vi "Logging2File.vi"(0 "log":string) -> (1 "LogFilePath":path, 2 "TimedLog":string)   [LabVIEW 2020]
doc: "Write to Log file and Send message to message window.\nLogs: .\\logs\\txt\nmessage: main.vi\\msg"
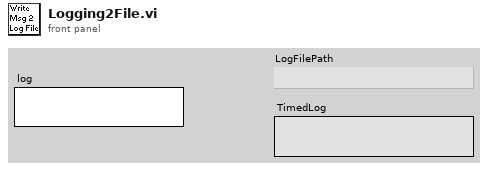
[diagram p1: front panel]
types:
  T1 = enum16{"open", "replace", "create", "open or create", "replace or create", "replace or create with confirmation"}
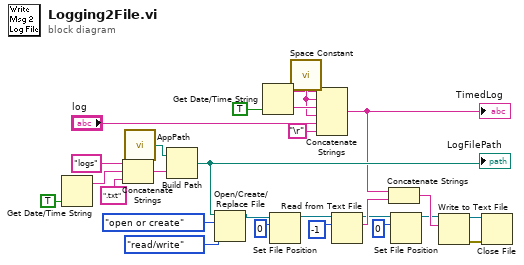
[diagram p0: block diagram]
diagram:
  n1 = Get Date/Time String(want seconds? (F)=TRUE) -> (date string=w24:string)  [unwired: 3 out]
  n2 = Concatenate Strings("logs" ("string"), w24, ".txt" ("string")) -> (w21:string)
  n3 = call "AppPath.vi"() -> ("AppPath"=w19:path)
  n4 = Build Path(base path=w19, name or relative path=w21) -> (appended path=w20:path)
  "LogFilePath" <- w20
  n5 = Open/Create/Replace File(file path (use dialog)=w20, operation (0:open)=T1."open or create", access (0:read/write)=enum16{"read/write", "read-only", "write-only"}."read/write") -> (refnum out=w1:refnum<file>)  [unwired: 1 in, 4 out]
  n6 = Get Date/Time String(want seconds? (F)=TRUE) -> (date string=w15:string, time string=w18:string)  [unwired: 2 out]
  n7 = Set File Position(offset (in bytes) (0)=i64 0, refnum=w1) -> (refnum out=w9:refnum<file>)  [unwired: 2 in, 1 out]
  n8 = call <vilib>:"Space Constant.vi"() -> ("String"=w17:string)
  n9 = Concatenate Strings(w15, w17, w18, w17, "log", "\r") -> (w4:string)
  "TimedLog" <- w4
  n10 = Read from Text File(file (use dialog)=w9, count=-1) -> (refnum out=w7:refnum<file>, text=w11:string)  [unwired: 2 in, 2 out]
  n11 = Concatenate Strings(w4, w11) -> (w12:string)
  n12 = Set File Position(offset (in bytes) (0)=i64 0, refnum=w7) -> (refnum out=w6:refnum<file>)  [unwired: 2 in, 1 out]
  n13 = Write to Text File(file (use dialog)=w6, text=w12) -> (refnum out=w2:refnum<file>, error out=w3:errorcluster)  [unwired: 2 in, 1 out]
  n14 = Close File(refnum=w2, error in=w3) -> ()  [unwired: 2 out]
